vi "Add New Line.vi"(8 "error in":errorcluster, 11 "objects":T1) -> (0 "error out":errorcluster, 1 "success":bool, 2 "Line Index":i32)   [LabVIEW 2014, in "PL Framework Configuration Tool.lvlib" / "Missing Plugin editor node.lvclass"]
doc: "This VI is called to add new elements to the configuration. \nIt creates a new default line and the opens the dialog to edit its properties. \nFinally it adds it to the configuration."
uses:
  Missing Plugin editor node.lvclass
  <vilib>/NI/DCAF/Tag Editor Core/Table API/Table Manager/object ref.ctl
  Engine Parent/Engine Parent Editor Node.lvclass
  Module editor node/module editor node.lvclass
  <vilib>/NI/DCAF/Tag Editor Core/Table API/Table Manager/Table Manager.lvclass
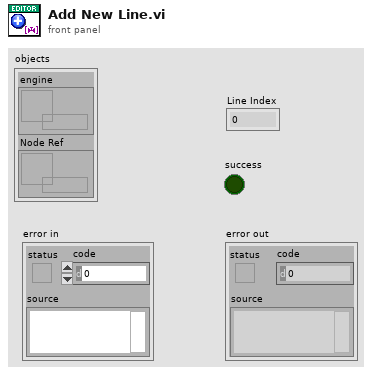
[diagram p1: front panel]
types:
  T1 = typedef "Table Manager.lvlib/Table Manager.lvclass/object ref.ctl" = cluster{"engine":refnum<data-value>, "Node Ref":refnum<data-value>}
  T2 = typedef "PL Framework Configuration Tool.lvlib/Missing Plugin configuration.lvclass/Line.ctl" = cluster{"channel":refnum<class "TBM channel.lvclass">}
  T3 = typedef "PL Framework Configuration Tool.lvlib/Missing Plugin editor node.lvclass/Mappings.ctl" = cluster{"Line":T2, "Maps":T4[]}
  T4 = typedef "PL Framework Configuration Tool.lvlib/Missing Plugin editor node.lvclass/Map.ctl" = cluster{"channel":refnum<class "TBM channel.lvclass">, "tag name":string}
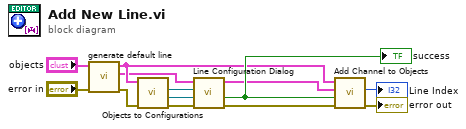
[diagram p0: block diagram]
diagram:
  n1 = call "generate default line.vi"("error in"="error in", "objects in"="objects") -> ("error out"=w4:errorcluster, "Line"=w5:T2, "objects out"=w8:T1)  [unwired: 7 in]
  n2 = call "Objects to Configurations.vi"("error in (no error)"=w4, "Objects in"=w8) -> ("error out"=w7:errorcluster, "engine configuration out"=w2:refnum<class "engine configuration.lvclass">, "tag bus configurable plugin module configuration"=w3:refnum<class "Missing Plugin configuration.lvclass">)  [unwired: 7 in]
  n3 = call "Line Configuration Dialog.vi"("error in"=w7, "engine configuration in"=w2, "tag bus configurable plugin module configuration"=w3, "Line"=w5) -> ("error out"=w11:errorcluster, "success"=w9:bool, "Mappings out"=w6:T3)  [unwired: 4 in, 1 out]
  "success" <- w9
  n4 = call "Add Channel to Objects.vi"("error in"=w11, "Add? (T)"=w9, "Line Item in"=w6, "Objects in"=w8) -> ("error out"=→"error out":errorcluster, "Line Index"=→"Line Index":i32)  [unwired: 6 in]
